vi "InitializeSoundCard.vi"(2 "Settings.Labels":string[](array[string])=["Hammer (V)", "Microphone (V)"], 3 "DeviceXControl":T1={"device ID"=0, "Device Name"="", "number of samples/ch"=0, "sample mode"=1, "sound format"={"sample rate (S/s)"=22050.0, "number of channels"=2, "bits per sample"=16}, "Sample length (sec)"=0.5, "Pre-trigger (sec)"=0.1} {"Pre-trigger (sec)" min=0.0 max=32.0 step=0.1 format="%#_4f"; "Sample length (sec)" min=0.0 max=32.0 step=0.1 format="%#_4f"; "sample mode" items=["Finite Samples", "Continuous Samples"]}) -> (1 "All Info":T4 {"Data Set"."Settings"."Time" format="%<%H:%M\n%d/%m/%y>T"; "task ID" format="%.0x"})   [LabVIEW 2014]
uses:
  <userlib>/CurtinCode/AllDataCtrl.ctl
  <userlib>/CurtinCode/DataControl.ctl
  <userlib>/CurtinCode/SettingsControl.ctl
  <vilib>/sound2/lvsound2.llb/Sound Input Task ID.ctl
  <userlib>/CurtinCode/Devicectrl/DeviceData.ctl
  <vilib>/sound2/lvsound2.llb/Sampling Mode.ctl
  <vilib>/sound2/lvsound2.llb/Sound Data Format.ctl
  <vilib>/DAQmx/create/channels.llb/DAQmx Create Channel (TEDS-AI-Sound Pressure-Microphone).vi
  <vilib>/DAQmx/create/channels.llb/DAQmx Create Channel (AI-Voltage-Basic).vi
  <vilib>/DAQmx/configure/timing.llb/DAQmx Timing (Sample Clock).vi
  <userlib>/CurtinCode/Devicectrl/Audio Channel.xctl
panel:
  out "number of samples/ch":i32=10000
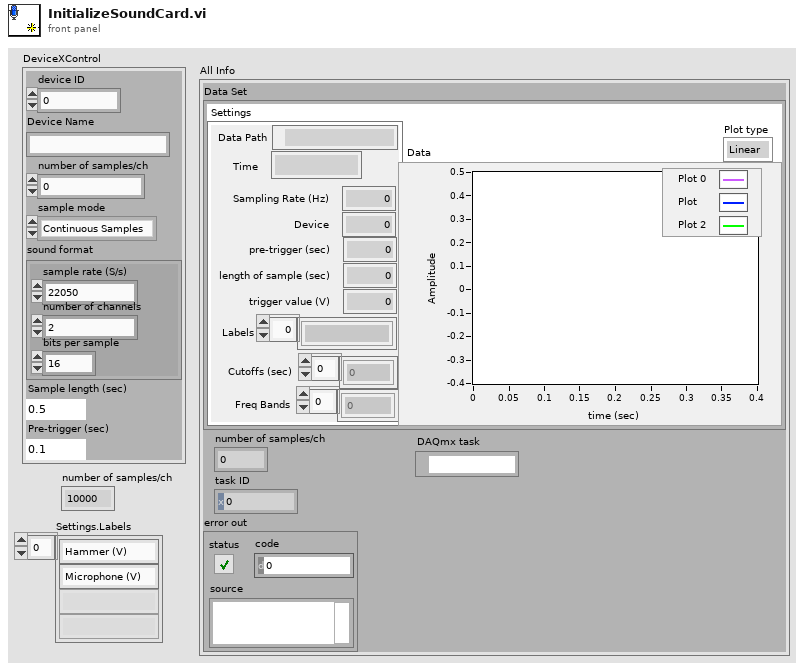
[diagram p1: front panel]
types:
  T1 = typedef "Audio Channel.xctl/DeviceData.ctl" = cluster{"device ID":u32, "Device Name":string, "number of samples/ch":i32, "sample mode":T2, "sound format":T3, "Sample length (sec)":dbl, "Pre-trigger (sec)":dbl}
  T2 = typedef "Sampling Mode.ctl" = i32
  T3 = typedef "Sound Data Format.ctl" = cluster{"sample rate (S/s)":dbl, "number of channels":i32, "bits per sample":i32}
  T4 = typedef "AllDataCtrl.ctl" = cluster{"Data Set":T5, "number of samples/ch":i32, "task ID":T7, "error out":errorcluster, "DAQmx task":refnum<k21>}
  T5 = typedef "DataControl.ctl" = cluster{"Settings":T6, "Data":cluster{i32, dbl, "data":dbl[]}[], "Plot type":enum16{"Linear", "log"}}
  T6 = typedef "SettingsControl.ctl" = cluster{"Data Path":path, "Time":timestamp, "Sampling Rate (Hz)":u16, "Device":u16, "pre-trigger (sec)":dbl, "length of sample (sec)":dbl, "trigger value (V)":dbl, "Labels":string[], "Cutoffs (sec)":dbl[], "Freq Bands":dbl[]}
  T7 = typedef "Sound Input Task ID.ctl" = u32
  T8 = cluster{"Data Set":T5, i32, "task ID":T7, "error out":errorcluster, "task out":refnum<k21>}
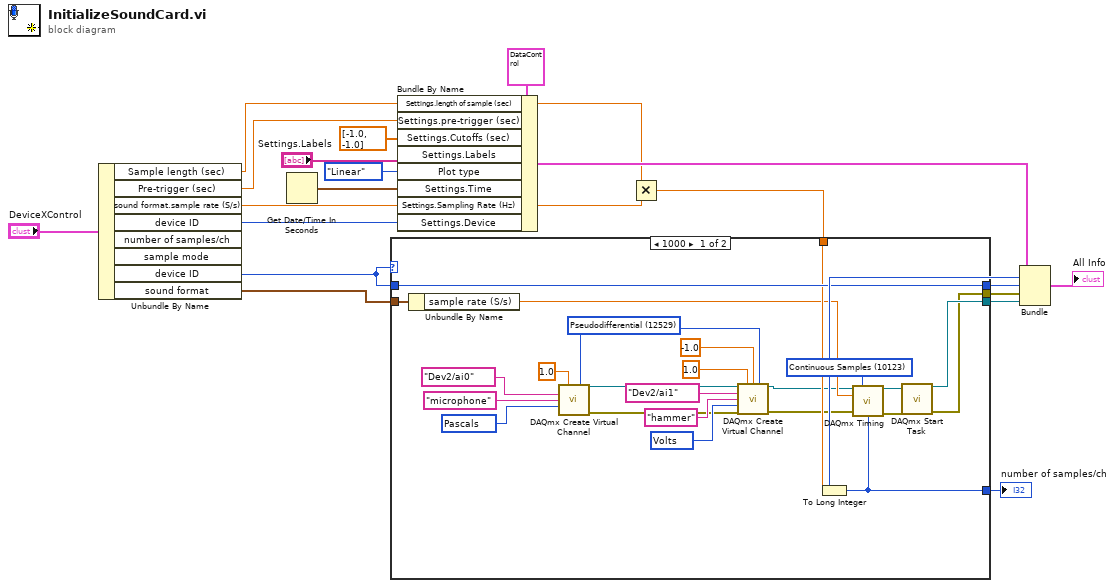
[diagram p0: block diagram]
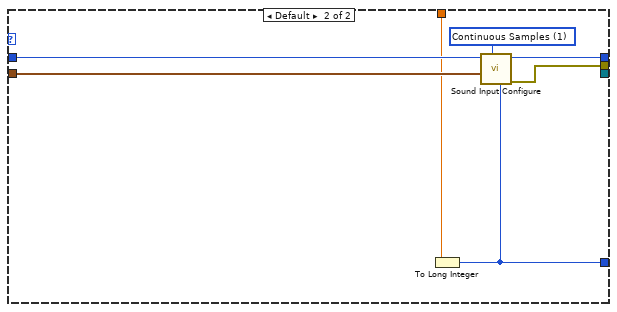
[diagram p2: hidden frame]
diagram:
  n1 = Unbundle By Name("DeviceXControl") -> ("Sample length (sec)"=w5:dbl, "Pre-trigger (sec)"=w4:dbl, "sound format.sample rate (S/s)"=w7:dbl, "device ID"=w12:u32, "device ID"=w2:u32, "sound format"=w10:T3)  [unwired: 2 out]
  n2 = Get Date/Time In Seconds() -> (seconds since 1Jan1904=w13:timestamp)
  n3 = Bundle By Name(cluster=T5 {"Settings"={"Data Path"=path "", "Time"=timestamp(0 s since 1904-01-01), "Sampling Rate (Hz)"=44800, "Device"=0, "pre-trigger (sec)"=100.0, "length of sample (sec)"=1000.0, "trigger value (V)"=100.0, "Labels"=[], "Cutoffs (sec)"=[], "Freq Bands"=[]}, "Data"=[], "Plot type"=enum."Linear"} ("Data Set"), "Settings.length of sample (sec)"=w5, "Settings.pre-trigger (sec)"=w4, "Settings.Cutoffs (sec)"=dbl[] [-1.0, -1.0] ("Settings.Cutoffs (V)"), "Settings.Labels"="Settings.Labels", "Plot type"=enum16{"Linear", "log"}."Linear", "Settings.Time"=w13, "Settings.Sampling Rate (Hz)"=w7, "Settings.Device"=w12) -> (w16:T5)
  n4 = Multiply(x=w5, y=w7) -> (x*y=w6:dbl)
  n5 = case shown="1000" w2 {
    tunnel: [w24 w50] -> w18
    tunnel: [w43 w49] -> w17
    tunnel: w10 -> [w29 w47]
    tunnel: w2 -> [w43 w46]
    tunnel: w6 -> [w42 w45]
    tunnel: [w30 w44] -> w3
    tunnel: [w25 _] -> w1
    frame 1000 {
      w40 = 10123 items=["Finite Samples"=10178, "Continuous Samples"=10123, "Hardware Timed Single Point"=12522] ("sample mode")
      w41 = 12529 items=["default"=-1, "RSE"=10083, "NRSE"=10078, "Differential"=10106, "Pseudodifferential"=12529] ("input terminal configuration")
      w36 = 10348 items=["Volts"=10348, "From Custom Scale"=10065] ("units")
      w32 = 10081 items=["Pascals"=10081, "From Custom Scale"=10065] ("units")
      n6 = Unbundle By Name(w29) -> ("sample rate (S/s)"=w28:dbl)
      n7 = call-poly <vilib>:"DAQmx Create Virtual Channel.vi"("maximum sound pressure level"=1.0, "input terminal configuration"=w41, "physical channels"=tag "Dev2/ai0", "name to assign"="microphone", "units"=w32) -> ("task out"=w23:refnum<k21>, "error out"=w20:errorcluster)  [unwired: 9 in]
      n8 = call-poly <vilib>:"DAQmx Create Virtual Channel.vi"("task in"=w23, "maximum value"=1.0, "minimum value"=-1.0, "input terminal configuration"=w41, "physical channels"=tag "Dev2/ai1", "name to assign"="hammer", "units"=w36, "error in"=w20) -> ("task out"=w22:refnum<k21>, "error out"=w21:errorcluster)  [unwired: 6 in]
      n9 = To Long Integer(number=w42) -> (32bit integer=w30:i32)
      n10 = call-poly <vilib>:"DAQmx Timing.vi"("task/channels in"=w22, "sample mode"=w40, "samples per channel"=w30, "rate"=w28, "error in"=w21) -> ("task out"=w27:refnum<k21>, "error out"=w26:errorcluster)  [unwired: 9 in]
      n11 = call <vilib>:"DAQmx Start Task.vi"("task/channels in"=w27, "error in"=w26) -> ("task out"=w25:refnum<k21>, "error out"=w24:errorcluster)  [unwired: 12 in]
    }
    frame Default {
      w48 = T2 1 items=["Finite Samples", "Continuous Samples"] ("sample mode")
      n12 = To Long Integer(number=w45) -> (32bit integer=w44:i32)
      n13 = call <vilib>:"Sound Input Configure.vi"("number of samples/ch"=w44, "sample mode"=w48, "sound format"=w47, "device ID"=w46) -> ("error out"=w50:errorcluster, "task ID"=w49:T7)  [unwired: 6 in]
    }
  }
  "number of samples/ch" <- w3
  n14 = Bundle("Data Set"=w16, w3, "task ID"=w17, "error out"=w18, "task out"=w1) -> (→"All Info":T8)  [unwired: 1 in]
